vi "Write-Read String Demo.vi"() -> ()   [LabVIEW 2016]
panel:
  out "error out":errorcluster
  in  "Flow Control":u16(ring) items=["None"=0, "RTS-CTS"=256, "DTR-DSR"=512, "XOn-XOff"=1024]
  in  "Parity":u8(ring) items=["FT_PARITY_NONE", "FT_PARITY_ODD", "FT_PARITY_EVEN", "FT_PARITY_MARK", "FT_PARITY_SPACE"]
  in  "Stop Bits":u8(ring) items=["FT_STOP_BITS_1"=0, "FT_STOP_BITS_2"=2]
  in  "Word Length":u8(ring)=8 items=["FT_BITS_7"=7, "FT_BITS_8"=8]
  in  "Baud Rate":u32=115200
  out "Read Buffer Out":string
  in  "Buffer":string="MATRIX.TEMPERATURE"
  out "Bytes Written":u32
  out "Device Description":string
  in  "Device Index":u32
  out "Bytes Read":u32
  out "Bytes Waiting":u32
  # "Enter values in Write Buffer and run program.  \nWith a loop-back connector, the data is read back into the Read Buffer."
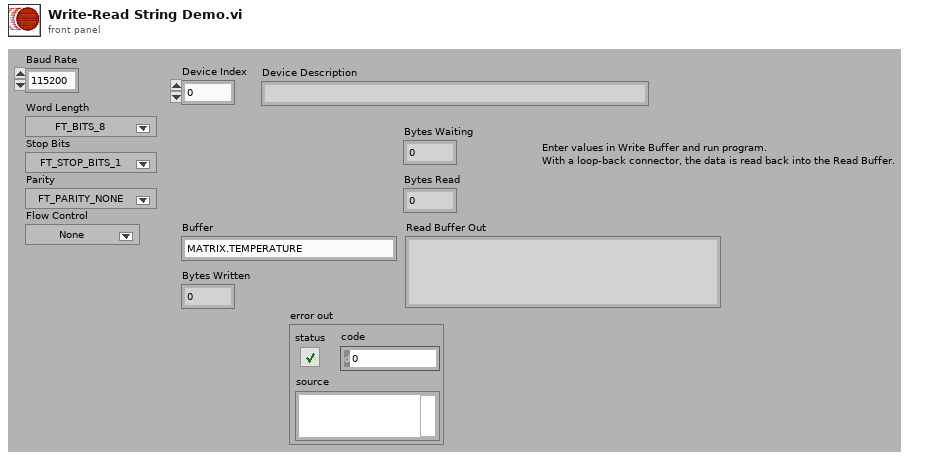
[diagram p1: front panel]
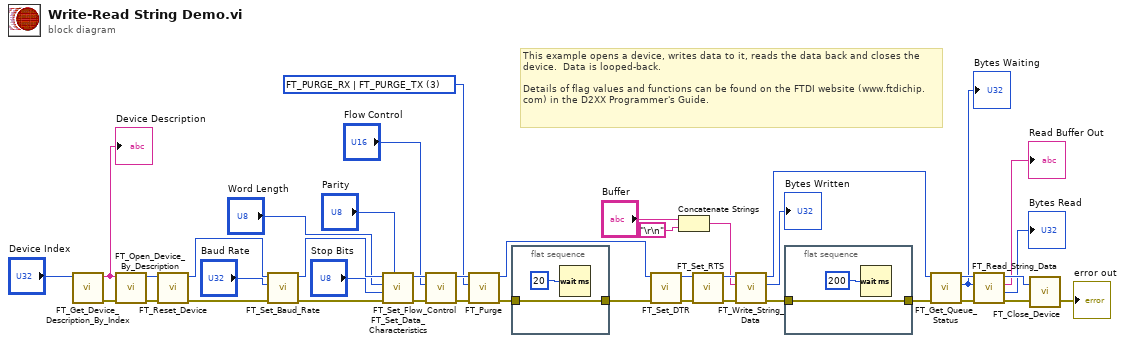
[diagram p0: block diagram]
diagram:
  w22 = u32 3 items=["FT_PURGE_RX"=1, "FT_PURGE_TX"=2, "FT_PURGE_RX | FT_PURGE_TX"=3] ("Purge Flags")
  # "This example opens a device, writes data to it, reads the data back and closes the device.  Data is looped-back.\n\nDetails of flag values and functions can be found on the FTDI website (www.ftdichip.com) in the D2XX Programmer's Guide."
  n1 = call "FT_Get_Device_Description_By_Index.vi"("Device Index"="Device Index") -> ("error out"=w8:errorcluster, "Device Description"=w41:string)  [unwired: 9 in]
  "Device Description" <- w41
  n2 = call "FT_Open_Device_By_Description.vi"("error in"=w8, "Device Description"=w41) -> ("error out"=w7:errorcluster, "Handle"=w40:u32)  [unwired: 8 in]
  n3 = call "FT_Reset_Device.vi"("error in"=w7, "Handle"=w40) -> ("error out"=w6:errorcluster, "Handle out"=w39:u32)  [unwired: 8 in]
  n4 = call "FT_Set_Baud_Rate.vi"("error in"=w6, "Baud Rate"="Baud Rate", "Handle"=w39) -> ("error out"=w5:errorcluster, "Handle out"=w38:u32)  [unwired: 7 in]
  n5 = call "FT_Set_Data_Characteristics.vi"("Parity"="Parity", "error in"=w5, "Stop Bits"="Stop Bits", "Word Length"="Word Length", "Handle"=w38) -> ("error out"=w4:errorcluster, "Handle out"=w37:u32)  [unwired: 5 in]
  n6 = call "FT_Set_Flow_Control.vi"("error in"=w4, "Flow Control"="Flow Control", "Handle"=w37) -> ("error out"=w3:errorcluster, "Handle out"=w36:u32)  [unwired: 7 in]
  n7 = call "FT_Purge.vi"("error in"=w3, "Purge Flags"=w22, "Handle"=w36) -> ("error out"=w15:errorcluster, "Handle out"=w35:u32)  [unwired: 7 in]
  n8 = flat-sequence {
    tunnel: w15 -> [w42]
    tunnel: [w42] -> w14
    frame #0 {
      n9 = Wait (ms)(milliseconds to wait=u32 20) -> ()  [unwired: 1 out]
    }
  }
  n10 = call "FT_Set_DTR.vi"("error in"=w14, "Handle"=w35) -> ("error out"=w2:errorcluster, "Handle out"=w34:u32)  [unwired: 8 in]
  n11 = Concatenate Strings("Buffer", "\r\n") -> (w19:string)
  n12 = call "FT_Set_RTS.vi"("error in"=w2, "Handle"=w34) -> ("error out"=w1:errorcluster, "Handle out"=w33:u32)  [unwired: 8 in]
  n13 = call "FT_Write_String_Data.vi"("error in"=w1, "Buffer"=w19, "Handle"=w33) -> ("error out"=w13:errorcluster, "Bytes Written"=→"Bytes Written":u32, "Handle out"=w32:u32)  [unwired: 6 in]
  n14 = flat-sequence {
    tunnel: [w44] -> w12
    tunnel: w13 -> [w44]
    frame #0 {
      n15 = Wait (ms)(milliseconds to wait=u32 200) -> ()  [unwired: 1 out]
    }
  }
  n16 = call "FT_Get_Queue_Status.vi"("error in"=w12, "Handle"=w32) -> ("error out"=w11:errorcluster, "Bytes Waiting"=w29:u32, "Handle out"=w31:u32)  [unwired: 7 in]
  "Bytes Waiting" <- w29
  n17 = call "FT_Read_String_Data.vi"("error in"=w11, "Bytes To Read"=w29, "Handle"=w31) -> ("error out"=w10:errorcluster, "Bytes Read"=→"Bytes Read":u32, "Read Data"=→"Read Buffer Out":string, "Handle out"=w30:u32)  [unwired: 5 in]
  n18 = call "FT_Close_Device.vi"("error in"=w10, "Handle"=w30) -> ("error out"=→"error out":errorcluster)  [unwired: 1 out]
